vi "XIPIN_Fixed_Interval_Timer_2_0.vi"   [LabVIEW 2017]
doc: "Generates an interrupt periodically\n------------------------------------\n<b>Need License</b> : No"
uses:
  <vilib>/rvi/XilinxIP/XIPIN_XNode/niFpgaXIPIN.xnode
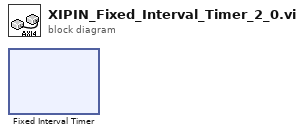
[diagram p0: block diagram]
diagram:
  n1 = xnode ("Fixed Interval Timer")() -> ()
